vi "Rebuild Boards Table.vi"() -> ()   [LabVIEW 2019, in "LINXx.lvlib"]
doc: "Dev helper to automatically generate table of supported boards from the firmware"
uses:
  LINXx.lvlib
panel:
  out "String":string
  in  "Regen LINX  instead?":bool
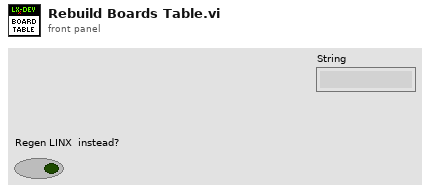
[diagram p1: front panel]
types:
  T1 = enum16{"open", "replace", "create", "open or create", "replace or create", "replace or create with confirmation"}
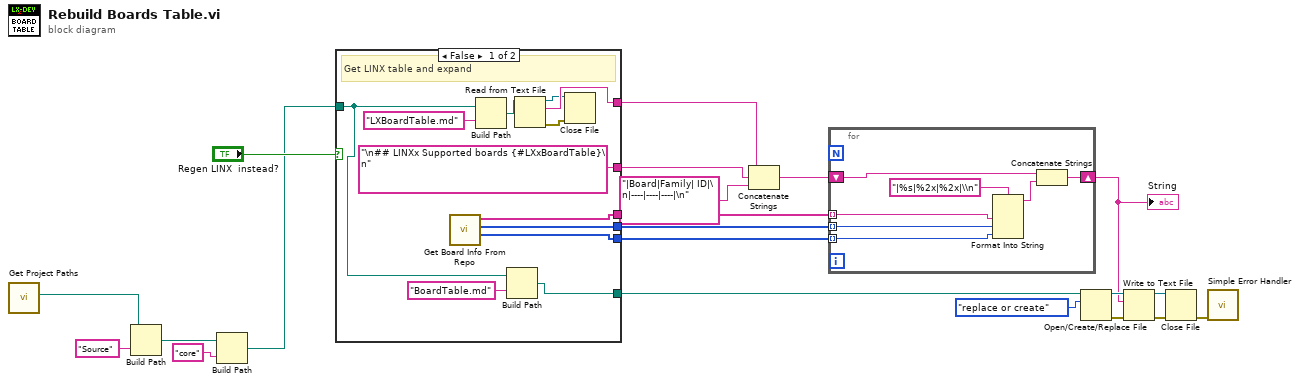
[diagram p0: block diagram]
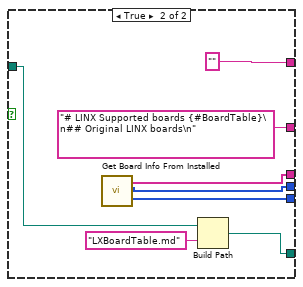
[diagram p2: hidden frame]
diagram:
  n1 = call "Get Project Paths.vi"() -> ("Firmware path"=w3:path)  [unwired: 8 in, 3 out]
  n2 = Build Path(base path=w3, name or relative path="Source") -> (appended path=w2:path)
  n3 = Build Path(base path=w2, name or relative path="core") -> (appended path=w1:path)
  n4 = case shown="False" "Regen LINX  instead?" {
    tunnel: ["\n## LINXx Supported boards {#LXxBoardTable}\n" "# LINX Supported boards {#BoardTable}\n## Original LINX boards\n"] -> w13
    tunnel: [w29 "" ("name or relative path")] -> w7
    tunnel: [w32 w37] -> w12
    tunnel: [w31 w38] -> w11
    tunnel: [w30 w39] -> w10
    tunnel: w1 -> [w22 w35]
    tunnel: [w23 w34] -> w6
    frame False {
      # "Get LINX table and expand"
      n5 = call "Get Board Info From Repo.vi"() -> ("Sorted ID"=w32:u32[], "Sorted Fam"=w31:u32[], "Sorted name"=w30:string[])  [unwired: 9 in]
      n6 = Build Path(base path=w22, name or relative path="LXBoardTable.md") -> (appended path=w25:path)
      n7 = Build Path(base path=w22, name or relative path="BoardTable.md") -> (appended path=w23:path)
      n8 = Read from Text File(file (use dialog)=w25) -> (refnum out=w27:refnum<file>, text=w29:string, error out=w28:errorcluster)  [unwired: 3 in, 1 out]
      n9 = Close File(refnum=w27, error in=w28) -> ()  [unwired: 2 out]
    }
    frame True {
      n10 = call "Get Board Info From Installed.vi"() -> ("Sorted ID"=w37:u32[], "Sorted Fam"=w38:u32[], "Sorted name"=w39:string[])  [unwired: 9 in]
      n11 = Build Path(base path=w35, name or relative path="LXBoardTable.md") -> (appended path=w34:path)
    }
  }
  n12 = Concatenate Strings(w7, w13, "|Board|Family| ID|\n|----|----|----|\n" ("string")) -> (w9:string)
  n13 = for {
    tunnel: w10 -> [w46] mode=indexing
    tunnel: w11 -> [w44] mode=indexing
    tunnel: w12 -> [w45] mode=indexing
    shift-right: [w42] -> w15
    shift-left: w9 -> [w48]
    n14 = Format Into String(format string="|%s|%2x|%2x|\\n", w46, w44, w45) -> (resulting string=w43:string)  [unwired: 2 in, 1 out]
    n15 = Concatenate Strings(w48, w43) -> (w42:string)
  }
  "String" <- w15
  n16 = Open/Create/Replace File(file path (use dialog)=w6, operation (0:open)=T1."replace or create") -> (refnum out=w19:refnum<file>, error out=w20:errorcluster)  [unwired: 4 in, 1 out]
  n17 = Write to Text File(file (use dialog)=w19, text=w15, error in=w20) -> (refnum out=w18:refnum<file>, error out=w21:errorcluster)  [unwired: 1 in, 1 out]
  n18 = Close File(refnum=w18, error in=w21) -> (error out=w16:errorcluster)  [unwired: 1 out]
  n19 = call <vilib>:"Simple Error Handler.vi"("error in (no error)"=w16) -> ()  [unwired: 4 in, 5 out]
